vi "Get Write Data to VS Channel Refs.vi"(8 "error in (no error)":errorcluster, 10 "Hardware Output Refs":T1[](array[typedef]) format="%.0x", 11 "Device Ref":T1 format="%.0x") -> (0 "error out":errorcluster, 2 "Write to VS Engine":cluster{"Refs":T2[], "Values":dbl[]} {"Refs" format="%.0x"}, 3 "Device Ref out":T1=18446744073709551615 format="%.0x")   [LabVIEW 2018, in "FPGA Addon System Explorer.lvlib"]
uses:
  FPGA Addon System Explorer.lvlib
  <vilib>/NI VeriStand/Custom Device API/Data Reference.ctl
  <vilib>/NI VeriStand/Custom Device API/Custom Device API.lvlib
  <vilib>/NI VeriStand/Custom Device API/Data Access Type.ctl
  <vilib>/NI VeriStand/Custom Device API/Custom Device Item Ref.ctl
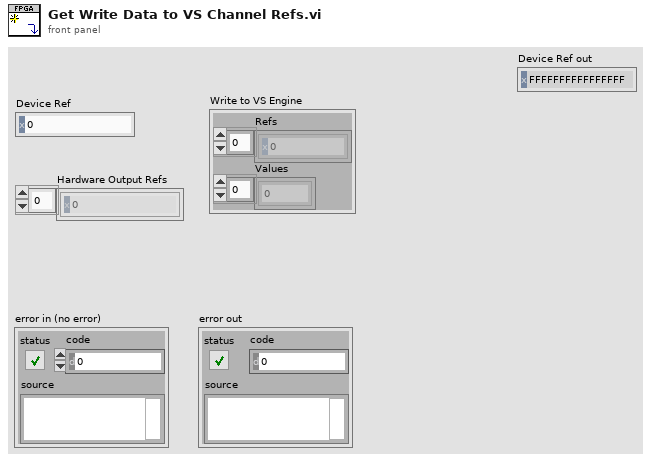
[diagram p1: front panel]
types:
  T1 = typedef "Custom Device API.lvlib/Custom Device Item Ref.ctl" = u64
  T2 = typedef "Custom Device API.lvlib/Data Reference.ctl" = i32
  T3 = typedef "Custom Device API.lvlib/Data Access Type.ctl" = enum16{"Read", "Write"}
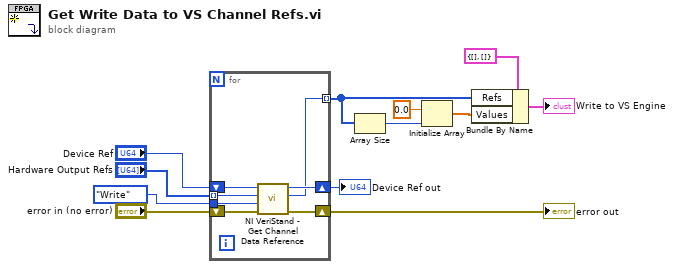
[diagram p0: block diagram]
diagram:
  n1 = for {
    tunnel: "Hardware Output Refs" -> [w15] mode=indexing
    tunnel: Data_Access_Type."Write" ("Access") -> [w14]
    shift-right: [w17] -> w1
    shift-left: "error in (no error)" -> [w18]
    shift-right: [w19] -> w3
    shift-left: "Device Ref" -> [w16]
    tunnel: [w13] -> w4 mode=indexing
    n2 = call <vilib>:"NI VeriStand - Get Channel Data Reference.vi"("error in (no error)"=w18, "Access"=w14, "Channel Ref in"=w15, "Device Ref in"=w16) -> ("error out"=w17:errorcluster, "Channel Data Reference"=w13:T2, "Device Ref out"=w19:T1)  [unwired: 5 in]
  }
  "error out" <- w1
  "Device Ref out" <- w3
  n3 = Array Size(array=w4) -> (size(s)=w9:i32)
  n4 = Initialize Array(0.0 ("element"), w9) -> (w11:dbl[])
  n5 = Bundle By Name(cluster=cluster{"Refs":T2[], "Values":dbl[]} {"Refs"=[], "Values"=[]} ("Write to VS Engine"), "Refs"=w4, "Values"=w11) -> (→"Write to VS Engine":cluster{"Refs":T2[], "Values":dbl[]})
